vi "CRYLimit edit global.vi"() -> ()   [LabVIEW 2013]
panel:
  out "RoundOff":bool
  out "ContinueF":bool
  out "Lower Limit":dbl
  out "Upper Limit":dbl
  out "Limits On":bool
  out "Lower Failed":cluster{dbl, dbl}[](array[cluster])
  out "Upper Failed":cluster{dbl, dbl}[](array[cluster])
  out "align ref point":cluster{dbl, dbl}[](array[cluster])
  out "critical point":cluster{dbl, dbl}[](array[cluster])
  out "Data":cluster{"x":dbl, "y":dbl}[](array[cluster])
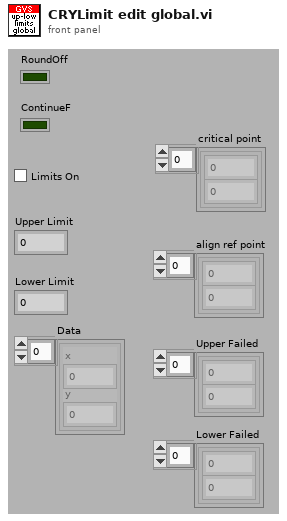
[diagram p1: front panel]
diagram:
